vi "colores.vi"() -> ()   [LabVIEW 2016]
panel:
  out "Color Box":u32(colorbox)
  in  "B":dbl(slide) scale=0.0..255.0
  in  "G":dbl(slide) scale=0.0..255.0
  in  "R":dbl(slide) scale=0.0..255.0
  in  "Stop Button":bool
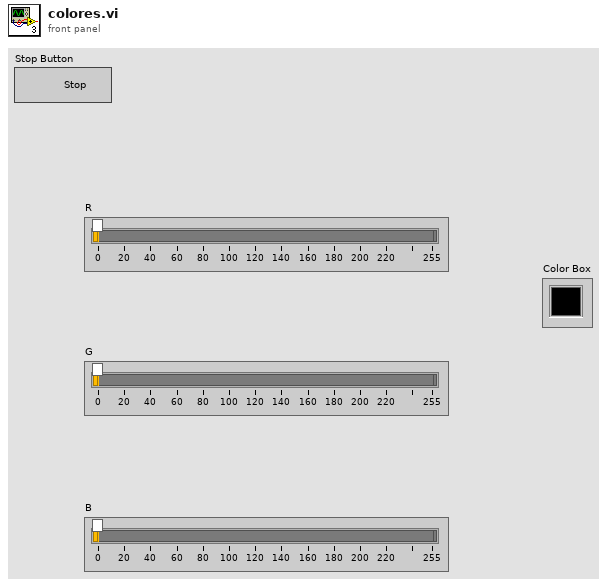
[diagram p1: front panel]
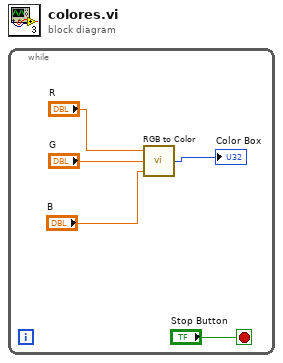
[diagram p0: block diagram]
diagram:
  n1 = while {
    stop <- "Stop Button" stop-if-true
    n2 = call <vilib>:"RGB to Color.vi"("B"="B", "G"="G", "R"="R") -> ("Color"=→"Color Box":u32)
  }
